vi "Get KFMparam from PGserver.vi"(6 "conninfo":T4={"host"="localhost", "port"="5432", "client_encoding"="WIN1251", "dbname"="data", "user"="postgres", "password"=""}, 8 "error in (no error)":errorcluster, 9 "KFMParamColumns":string[](array[string])=["MVIName", "ip_adress", "port", "connection_timeout", "reconnection_timeout", "n_attempt_max", "reset_connect_timeout", "write_timeout", "read_timeout", "period", "enable", "write_enable", "fcode_full"], 10 "KFMParamTable":string="kfm_3", 11 "KFMParameters":string[](array[string])) -> (0 "error out":errorcluster, 1 "timeouts":T1[](array[typedef]), 2 "IP Address":T2(array[cluster]), 3 "MVIName":string[](array[string]), 4 "enable":bool[][](array[boolean]))   [LabVIEW 2021]
uses:
  PostgreSQL/PostgreSQL2LabVIEW/ctl/Coninfo.ctl
  MBTCP Param/Typedefs/timeouts.ctl
  PostgreSQL/PostgreSQL2LabVIEW/libpqlv/src/PQfinish.vi
  PostgreSQL/PostgreSQL2LabVIEW/libpqlv/src/PQconnectdb.vi
  PostgreSQL/PostgreSQL2LabVIEW/libpqlv/src/PQerrorMessage.vi
  PostgreSQL/PostgreSQL2LabVIEW/libpqlv/src/PQstatus.vi
  <vilib>/dlg_ctls.llb/Space Constant.vi
  PostgreSQL/PostgreSQL2LabVIEW/libpqUtility/libpqutility.lvlib
  MBTCP Param/MBTCP Param.lvclass
  PostgreSQL/PostgreSQL.lvlib
panel:
  out "progress 3":i32
  out "PQStatus":T3(ring)
  # "fcode_full"
  # "fname"
  # "process_unit"
  # "port"
  # "connection_timeout"
  # "n_attempt_max"
  # "process_low_acd"
  # "instrument_range_max"
  # "d"
  # "input_register_min"
  # "input_register_max"
  # "input_pv_min"
  # "input_pv_max"
  # "ip_adress"
  # "fcodef"
  # "instrument_max_offset"
  # "reconnection_timeout"
  # "control_channel_num"
  # "process_range_max"
  # "process_high_acd"
  # "process_high_alr"
  # "process_low_alr"
  # "module_num"
  # "MVIName"
  # "ip_adress"
  # "fcode"
  # "Names"
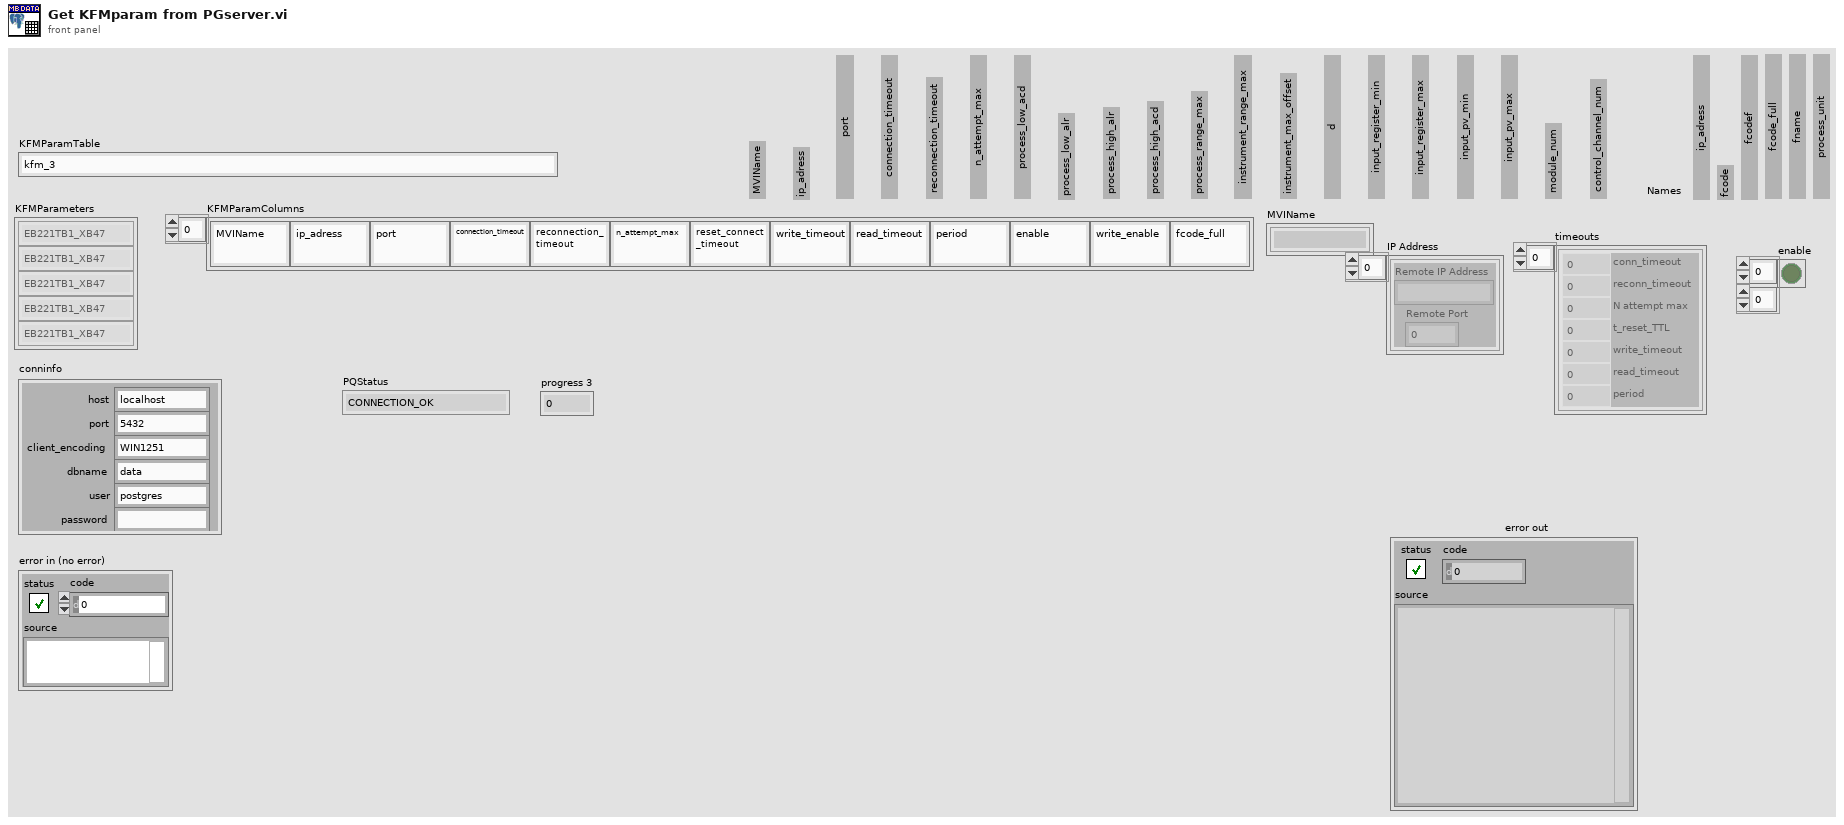
[diagram p1: front panel]
types:
  T1 = typedef "MBParam.lvlib/MBTCP Param.lvclass/timeouts.ctl" = cluster{"conn_timeout":i32, "reconn_timeout":i32, "N attempt max":i32, "t_reset_TTL":i32, "write_timeout":i32, "read_timeout":i32, "period":i32}
  T2 = cluster{"Remote IP Address":string, "Remote Port":u16}[]
  T3 = enum32{"CONNECTION_OK", "CONNECTION_BAD", "CONNECTION_STARTED", "CONNECTION_MADE", "CONNECTION_AWAITING_RESPONSE", "CONNECTION_AUTH_OK", "CONNECTION_SETENV", "CONNECTION_SSL_STARTUP", "CONNECTION_NEEDED"}
  T4 = typedef "libpqutility.lvlib/Coninfo.ctl" = cluster{"host":string, "port":string, "client_encoding":string, "dbname":string, "user":string, "password":string}
  T5 = cluster{"Remote IP Address":string, "Remote Port":u16}
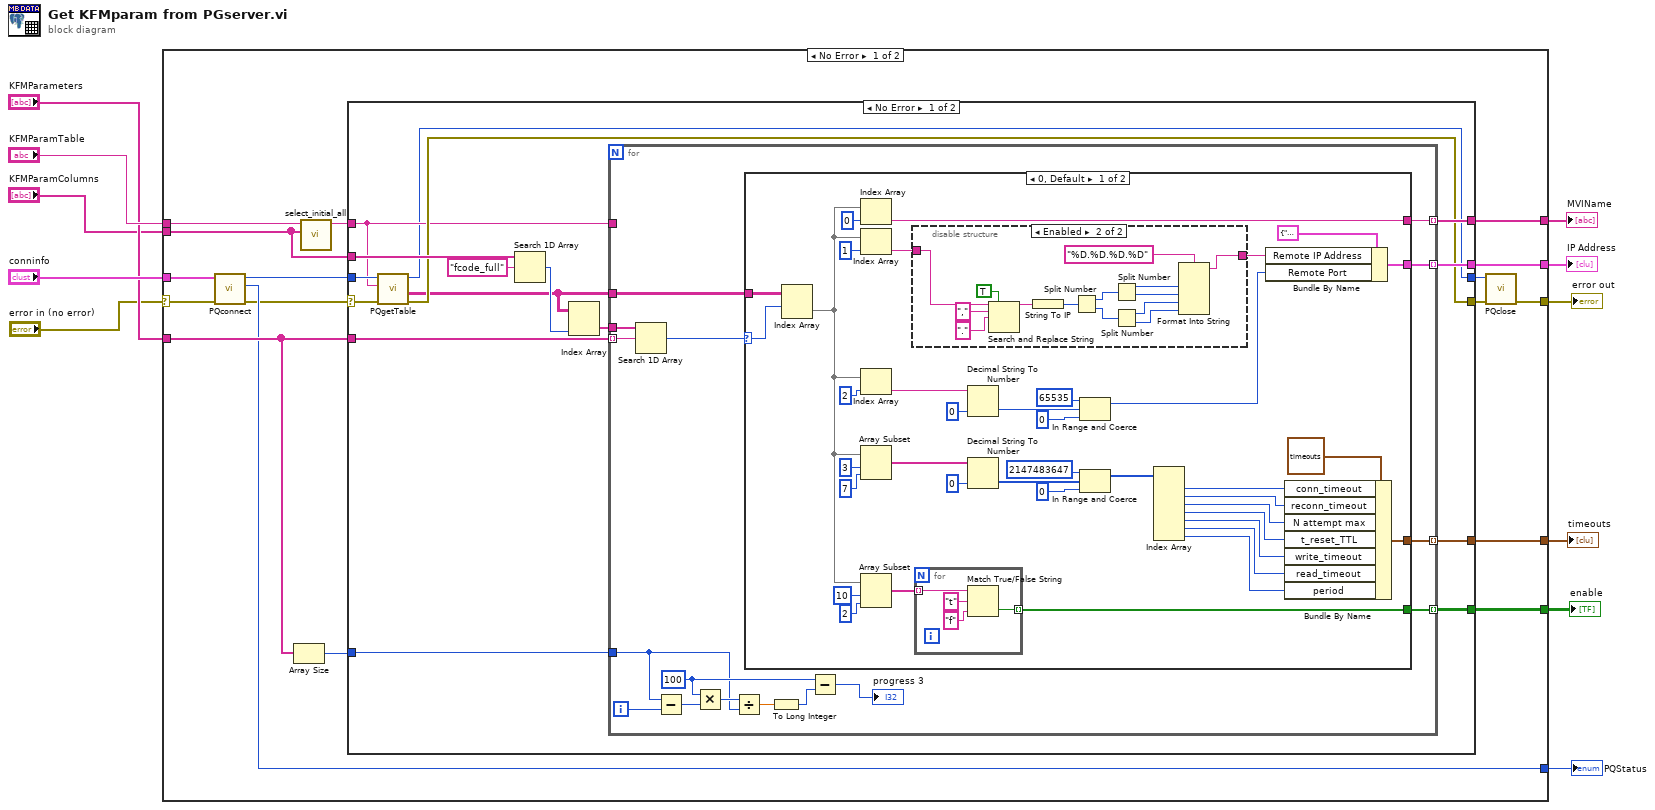
[diagram p0: block diagram]
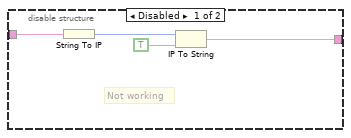
[diagram p2: hidden frame]
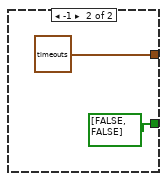
[diagram p3: hidden frame]
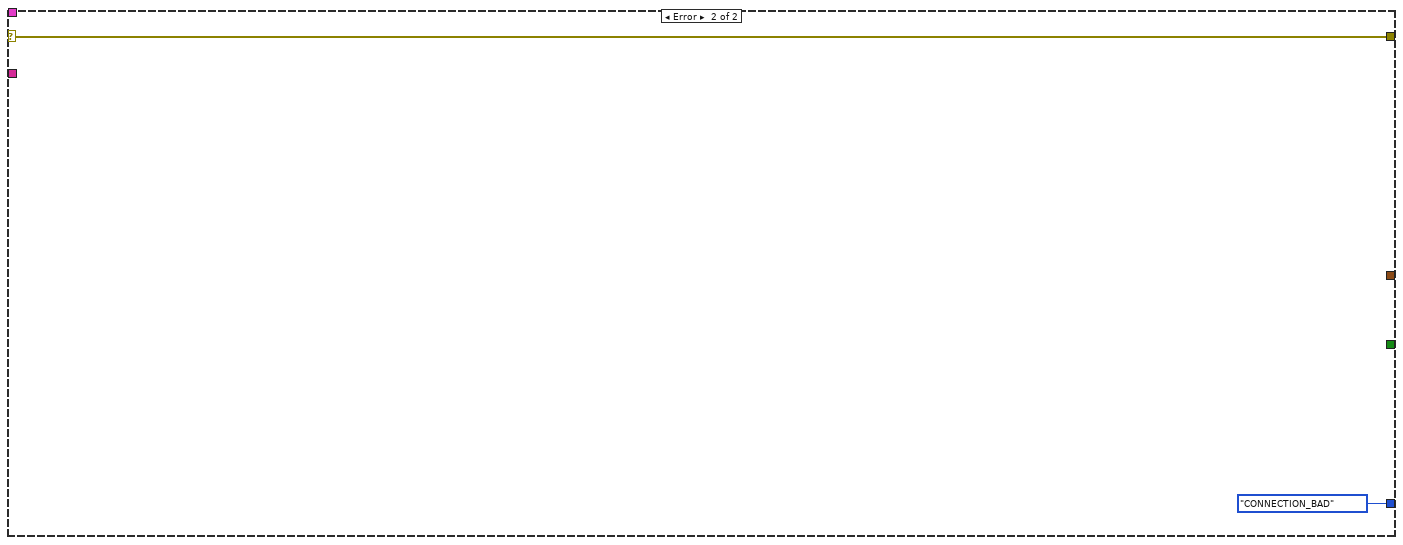
[diagram p5: hidden frame]
diagram:
  n1 = case shown="No Error" "error in (no error)" {
    selector: "error in (no error)" -> [w23 w126]
    tunnel: [w28 w126] -> w11
    tunnel: "KFMParamColumns" -> [w27 _]
    tunnel: "conninfo" -> [w26 _]
    tunnel: "KFMParamTable" -> [w25 _]
    tunnel: "KFMParameters" -> [w24 _]
    tunnel: [w22 T3."CONNECTION_BAD" ("PQStatus")] -> w6
    tunnel: [w21 _] -> w4
    tunnel: [w20 _] -> w3
    tunnel: [w19 _] -> w2
    tunnel: [w18 _] -> w1
    frame No Error {
      n2 = call "PQconnect.vi"("error in (no error)"=w23, "conninfo"=w26) -> ("error out"=w14:errorcluster, "PQStatus"=w22:T3, "conn"=w15:u64)  [unwired: 7 in]
      n3 = Array Size(array=w24) -> (size(s)=w17:i32)
      n4 = call "select_initial_all.vi"("Column table"=w27, "table"=w25) -> ("parameters"=w16:string)  [unwired: 8 in, 1 out]
      n5 = case shown="No Error" w14 {
        selector: w14 -> [w29 w124]
        tunnel: w24 -> [w43 _]
        tunnel: w17 -> [w44 _]
        tunnel: w15 -> [w33 w123]
        tunnel: w16 -> [w32 _]
        tunnel: [w34 w124] -> w13
        tunnel: [w31 w123] -> w12
        tunnel: [w42 _] -> w21
        tunnel: [w41 _] -> w20
        tunnel: [w40 _] -> w19
        tunnel: [w39 _] -> w18
        tunnel: w27 -> [w35 _]
        frame No Error {
          n6 = call "PQgetTable.vi"("error in"=w29, "query"=w32, "conn"=w33) -> ("error out"=w34:errorcluster, "Data"=w30:string[][], "conn_out"=w31:u64)  [unwired: 4 in, 2 out]
          n7 = Search 1D Array(1D array=w35, element="fcode_full" ("table")) -> (index of element=w37:i32)  [unwired: 1 in]
          n8 = Index Array(array=w30, index (col)=w37) -> (element=w36:string[])  [unwired: 1 in]
          n9 = for {
            tunnel: w44 -> [w54]
            tunnel: w43 -> [w46] mode=indexing
            tunnel: w32 -> [_]
            tunnel: [w52] -> w42 mode=indexing
            tunnel: [w51] -> w41 mode=indexing
            tunnel: [w50] -> w40 mode=indexing
            tunnel: [w49] -> w39 mode=indexing
            tunnel: w30 -> [w48]
            tunnel: w36 -> [w47]
            i -> [w55]
            w59 = 100 ("y")
            n10 = Search 1D Array(1D array=w47, element=w46) -> (index of element=w45:i32)  [unwired: 1 in]
            n11 = Subtract(x=w54, y=w55) -> (x-y=w58:i32)
            n12 = Multiply(x=w59, y=w58) -> (x*y=w60:i32)
            n13 = Divide(x=w60, y=w54) -> (x/y=w57:dbl)
            n14 = case shown="0, Default" w45 {
              selector: w45 -> [w65 _]
              tunnel: [w97 _] -> w52
              tunnel: [w79 bool[] [FALSE, FALSE]] -> w50
              tunnel: [w78 _] -> w51
              tunnel: [w68 T1 {"conn_timeout"=1000, "reconn_timeout"=3000, "N attempt max"=3, "t_reset_TTL"=120000, "write_timeout"=50, "read_timeout"=500, "period"=100} ("timeouts")] -> w49
              tunnel: w48 -> [w67 _]
              frame 0, Default {
                n15 = Index Array(array=w67, index (row)=w65) -> (element=w81:string[])  [unwired: 1 in]
                n16 = Index Array(array=w81, index=0) -> (element=w97:string)
                n17 = Index Array(array=w81, index=1) -> (element=w96:string)
                n18 = Index Array(array=w81, index=2) -> (element=w92:string)
                n19 = Array Subset(array=w81, index=3, length=7 ("y")) -> (w84:string[])
                n20 = Array Subset(array=w81, index=10, length=2) -> (w80:string[])
                n21 = disable-structure shown="Enabled" {
                  disable-tunnel: w96 -> [w102 w104]
                  disable-tunnel: [w101 w103] -> w90
                  frame Disabled {
                    # "Not working"
                    n22 = String To IP(1:w102) -> (0:w100:u32)
                    n23 = IP To String(1:TRUE ("dot notation? (F)"), 2:w100) -> (0:w101:string)
                  }
                  frame Enabled {
                    n24 = Search and Replace String(replace all?=TRUE ("replace all? (F)"), input string=w104, search string=",", replace string="." ("replace string (\"\")")) -> (result string=w106:string)  [unwired: 4 in, 3 out]
                    n25 = String To IP(1:w106) -> (0:w116:u32)
                    n26 = Split Number(x=w116) -> (hi(x)=w115:u16, lo(x)=w114:u16)
                    n27 = Split Number(x=w115) -> (hi(x)=w112:u8, lo(x)=w111:u8)
                    n28 = Split Number(x=w114) -> (hi(x)=w110:u8, lo(x)=w109:u8)
                    n29 = Format Into String(format string="%D.%D.%D.%D", w112, w111, w110, w109) -> (resulting string=w103:string)  [unwired: 2 in, 1 out]
                  }
                }
                n30 = for {
                  tunnel: w80 -> [w119] mode=indexing
                  tunnel: [w117] -> w79 mode=indexing
                  n31 = Match True/False String(2:"f" ("false string"), 3:"t" ("true string"), 4:w119) -> (0:w117:bool)  [unwired: 1 out]
                }
                n32 = Decimal String To Number(string=w92, default (0L)=0 ("default (0 I32)")) -> (number=w89:i32)  [unwired: 1 in, 1 out]
                n33 = Decimal String To Number(string=w84, default (0L)=0 ("default (0 I32)")) -> (number=w61:i32[])  [unwired: 1 in, 1 out]
                n34 = In Range and Coerce(upper limit=65535, x=w89, lower limit=0) -> (coerced(x)=w86:i32)  [unwired: 1 out]
                n35 = In Range and Coerce(upper limit=2147483647, x=w61, lower limit=0) -> (coerced(x)=w69:i32[])  [unwired: 1 out]
                n36 = Index Array(array=w69) -> (element #1=w76:i32, element #2=w75:i32, element #3=w74:i32, element #4=w73:i32, element #5=w72:i32, element #6=w71:i32, element #7=w70:i32)  [unwired: 7 in]
                n37 = Bundle By Name(cluster=T5 {"Remote IP Address"="", "Remote Port"=502} ("IP address"), "Remote IP Address"=w90, "Remote Port"=w86) -> (w78:T5)
                n38 = Bundle By Name(cluster=T1 {"conn_timeout"=1000, "reconn_timeout"=3000, "N attempt max"=3, "t_reset_TTL"=120000, "write_timeout"=50, "read_timeout"=500, "period"=100} ("timeouts"), "conn_timeout"=w76, "reconn_timeout"=w75, "N attempt max"=w74, "t_reset_TTL"=w73, "write_timeout"=w72, "read_timeout"=w71, "period"=w70) -> (w68:T1)
              }
              frame -1 {
              }
            }
            n39 = To Long Integer(number=w57) -> (32bit integer=w56:i32)
            n40 = Subtract(x=w59, y=w56) -> (x-y=→"progress 3":i32)
          }
        }
        frame Error {
        }
      }
      n41 = call "PQclose.vi"("error in (no error)"=w13, "conn"=w12) -> ("error out"=w28:errorcluster)  [unwired: 9 in]
    }
    frame Error {
    }
  }
  "error out" <- w11
  "PQStatus" <- w6
  "MVIName" <- w4
  "enable" <- w2
  "IP Address" <- w3
  "timeouts" <- w1
